vi "LCR Full Advanced Sequence.vi"() -> ()   [LabVIEW 2023]
doc: "Overview: This example demonstrates how to make sweep times faster by using LCR Advanced Sequence functions to change the frequency in a sequence. During the sequence, the channel steps through the predetermined set configurations (frequency in this example) without any interaction with the host system. The advantage of sequencing is that changes from one step in the sequence to the next are deterministic.\nThe program will perform an AC Voltage frequency sweep from Start Frequency to End Frequency. The sweep frequencies are an exponential sequence and the length of each of the sweeps is equal to the value in the Number Of Steps control."
uses:
  <instrlib>/niDCPower/nidcpower.llb/niDCPower Source Mode.ctl
  <instrlib>/niDCPower/nidcpower.llb/niDCPower Wait For Event - Event.ctl
  <instrlib>/niDCPower/nidcpower.llb/niDCPower Sequence Attribute Type.ctl
  <instrlib>/niDCPower/nidcpower.llb/niDCPower Create Advanced Sequence Step With Channels.vi
  <vilib>/Utility/file.llb/Write Delimited Spreadsheet (DBL).vi
panel:
  out "error out":errorcluster
  in  "Hardware timed Instrument Settings":T1(array[cluster])=[{"Instrument Mode"=1062, "LCR:AC Stimulus:Voltage Amplitude"=0.1, "LCR:AC Stimulus:Frequency"=1000.0, "Source:DC Voltage:Voltage Level"=0.0, "Source:DC Voltage:Current Limit"=0.0}, {"Instrument Mode"=1062, "LCR:AC Stimulus:Voltage Amplitude"=0.15, "LCR:AC Stimulus:Frequency"=2000.0, "Source:DC Voltage:Voltage Level"=0.0, "Source:DC Voltage:Current Limit"=0.0}, {"Instrument Mode"=1061, "LCR:AC Stimulus:Voltage Amplitude"=0.0, "LCR:AC Stimulus:Frequency"=0.0, "Source:DC Voltage:Voltage Level"=2.0, "Source:DC Voltage:Current Limit"=1e-06}, {"Instrument Mode"=1061, "LCR:AC Stimulus:Voltage Amplitude"=0.0, "LCR:AC Stimulus:Frequency"=0.0, "Source:DC Voltage:Voltage Level"=4.0, "Source:DC Voltage:Current Limit"=1e-05}, {"Instrument Mode"=1062, "LCR:AC Stimulus:Voltage Amplitude"=0.2, "LCR:AC Stimulus:Frequency"=2000.0, "Source:DC Voltage:Voltage Level"=0.0, "Source:DC Voltage:Current Limit"=0.0}] {"Instrument Mode" items=["SMU PS"=1061, "LCR"=1062, "E-Load"=1154]}
  in  "file path (use dialog)":path
  in  "LCR Short Compensation Enabled":bool
  in  "LCR Open Compensation Enabled":bool
  in  "Impedance Range":dbl=100.0 format="%_6p"
  in  "Cable Length":i32(ring)=1123 items=["0m"=1121, "NI Standard 1m"=1122, "NI Standard 2m"=1123, "NI Standard 4m"=1124, "Custom (Onboard Storage)"=1125, "Custom (As Configured)"=1126, "NI Standard Triaxial 1m"=1139, "NI Standard Triaxial 2m"=1140, "NI Standard Triaxial 4m"=1141]
  in  "LCR Custom Measurement Time Sec":dbl caption="LCR Custom \nMeasurement Time Sec" format="%_3p"
  in  "LCR Measurement Time":i32(ring)=1072 items=["Short"=1071, "Medium"=1072, "Long"=1073, "Custom"=1117]
  in  "LCR DC Bias Source":i32(ring)=1066 items=["Off"=1065, "Voltage"=1066, "Current"=1067]
  in  "Voltage Amplitude RMS":dbl=0.7 format="%_6p"
  out "Impendance vs Frequency":T2(graph) caption="Impedance vs DC Voltage"
  in  "Channel Name":string="0"
  in  "Resource Name":refnum<k15>="Dev1"
  # "Overview: This example demonstrates how to make sweep times faster by using LCR Advanced Sequence functions to change the frequency in a sequence. During the sequence, the channel steps through the predetermined set configurations (frequency in this example) without any interaction with the host system. The advantage of sequencing is that changes from one step in the sequence to the next are deterministic. The program will perform an AC Voltage frequency sweep from Start Frequency to End Frequency. The sweep frequencies are an exponential sequence and the length of each of the sweeps is equal to the value in the Number Of Steps control. \n\nThe Cable Length option of \"Custom (As Configured)\" is not supported in this example. Search ni.com for information about NI power supplies/SMUs and the NI-DCPower API.\n\nRequirements: NI-DCPower\nInstructions:\n1. Select the appropriate instrument in the Resource Name control.\n2. Configure the parameters of the sweeps.\n3. Configure the Cable Length to match your cabling setup.\n4. Run the VI."
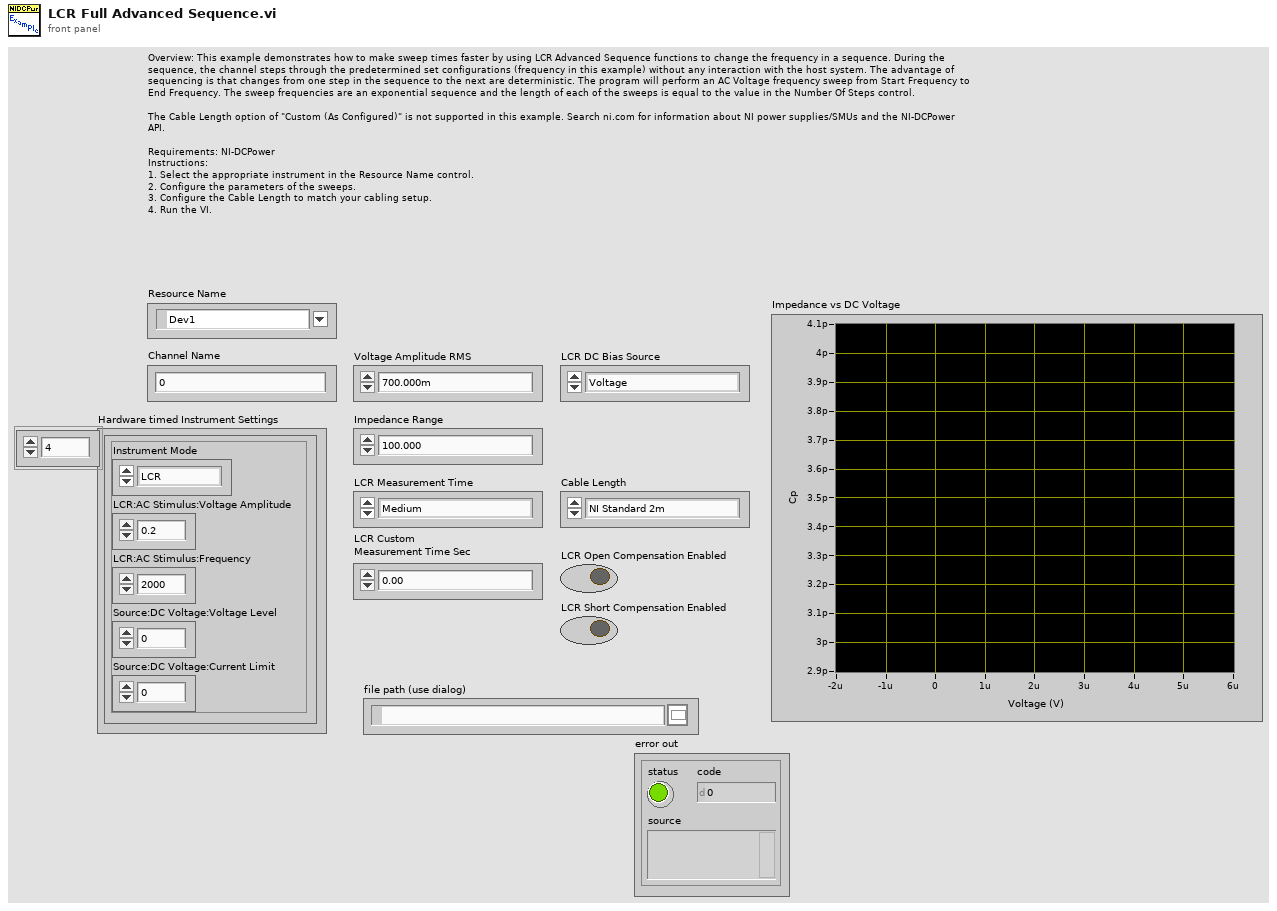
[diagram p1: front panel]
types:
  T1 = cluster{"Instrument Mode":i32, "LCR:AC Stimulus:Voltage Amplitude":dbl, "LCR:AC Stimulus:Frequency":dbl, "Source:DC Voltage:Voltage Level":dbl, "Source:DC Voltage:Current Limit":dbl}[]
  T2 = cluster{"voltage measurements":dbl[], "current measurements":dbl[]}
  T3 = typedef "niDCPower Sequence Attribute Type.ctl" = i32
  T4 = typedef "niDCPower Wait For Event - Event.ctl" = i32
  T5 = typedef "niDCPower Source Mode.ctl" = i32
  T6 = typedef "niDCPower LCR Measurement.ctl" = cluster{"V DC":dbl, "I DC":dbl, "stimulus frequency":dbl, "AC voltage":cdb, "AC current":cdb, "Z":cdb, "Z magnitude":dbl, "Z theta":dbl, "Y":cdb, "Y magnitude":dbl, "Y theta":dbl, "Ls":dbl, "Cs":dbl, "Rs":dbl, "Lp":dbl, "Cp":dbl, "Rp":dbl, "D":dbl, "Q":dbl, "measurement mode":u16, "DC in compliance":bool, "Pad 0":u8, "AC in compliance":bool, "Pad 1":u8, "unbalanced":bool, "Pad 2":u8, "Reserved 1":dbl, "Reserved 2":dbl, "Reserved 3":dbl, "Reserved 4":dbl, "Reserved 5":dbl, "Reserved 6":dbl, "Reserved 7":dbl}
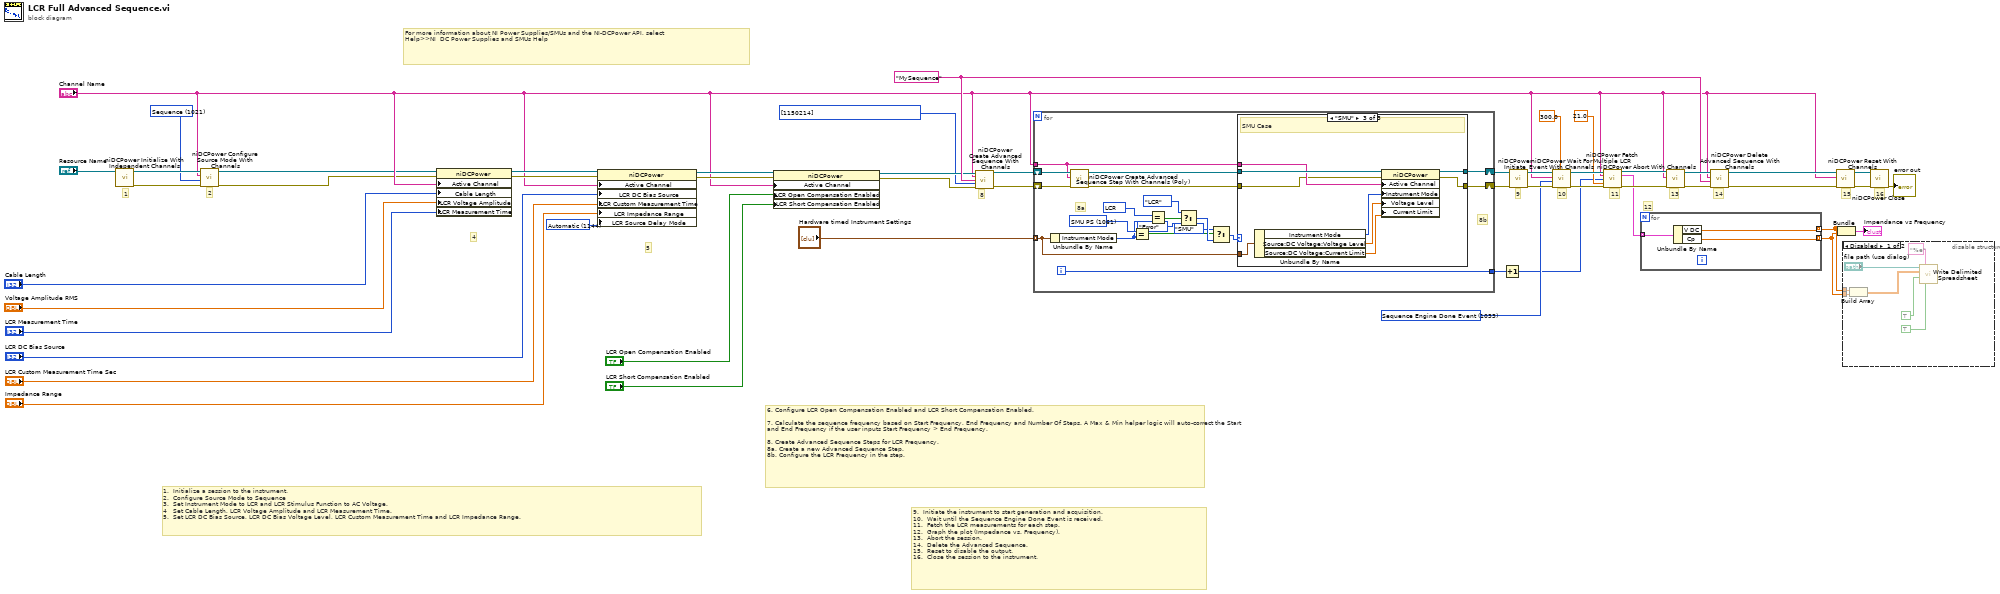
[diagram p0: block diagram]
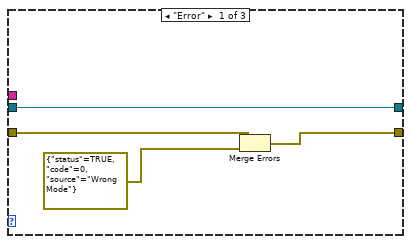
[diagram p3: hidden frame]
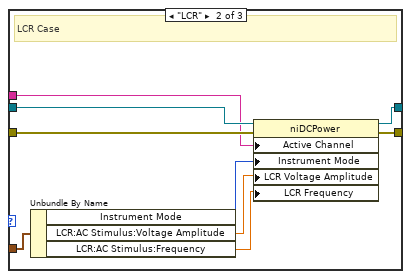
[diagram p4: hidden frame]
diagram:
  w11 = 1144 items=["Automatic"=1144, "Manual"=1145] ("LCR:Source Delay Mode")
  w12 = T3[] [1150214] items=["Source -> Output Function"=1150008, "Source -> Output Enabled"=1250006, "Source -> Output Resistance"=1150061, "Source -> Transient Response"=1150062, "Source -> Custom Transient Response -> Voltage Gain Bandwidth"=1150067, "Source -> Custom Transient Response -> Voltage Compensation Frequency"=1150068, "Source -> Custom Transient Response -> Voltage Pole-Zero Ratio"=1150069, "Source -> Custom Transient Response -> Current Gain Bandwidth"=1150070, "Source -> Custom Transient Response -> Current Compensation Frequency"=1150071, "Source -> Custom Transient Response -> Current Pole-Zero Ratio"=1150072, "Source -> DC Voltage -> Voltage Level"=1250001, "Source -> DC Voltage -> Voltage Level Range"=1150005, "Source -> DC Voltage -> Current Limit"=1250005, "Source -> DC Voltage -> Current Limit High"=1150187, "Source -> DC Voltage -> Current Limit Low"=1150188, "Source -> DC Voltage -> Current Limit Range"=1150004, "Source -> DC Current -> Current Level"=1150009, "Source -> DC Current -> Current Level Range"=1150011, "Source -> DC Current -> Voltage Limit"=1150010, "Source -> DC Current -> Voltage Limit High"=1150185, "Source -> DC Current -> Voltage Limit Low"=1150186, "Source -> DC Current -> Voltage Limit Range"=1150012, "Source -> Pulse Voltage -> Pulse Voltage Level"=1150080, "Source -> Pulse Voltage -> Pulse Bias Voltage Level"=1150082, "Source -> Pulse Voltage -> Pulse Voltage Level Range"=1150084, "Source -> Pulse Voltage -> Pulse Current Limit"=1150081, "Source -> Pulse Voltage -> Pulse Current Limit High"=1150193, "Source -> Pulse Voltage -> Pulse Current Limit Low"=1150194, "Source -> Pulse Voltage -> Pulse Bias Current Limit"=1150083, "Source -> Pulse Voltage -> Pulse Bias Current Limit High"=1150195, "Source -> Pulse Voltage -> Pulse Bias Current Limit Low"=1150196, "Source -> Pulse Voltage -> Pulse Current Limit Range"=1150085, "Source -> Pulse Current -> Pulse Current Level"=1150086, "Source -> Pulse Current -> Pulse Bias Current Level"=1150088, "Source -> Pulse Current -> Pulse Current Level Range"=1150090, "Source -> Pulse Current -> Pulse Voltage Limit"=1150087, "Source -> Pulse Current -> Pulse Voltage Limit High"=1150189, "Source -> Pulse Current -> Pulse Voltage Limit Low"=1150190, "Source -> Pulse Current -> Pulse Bias Voltage Limit"=1150089, "Source -> Pulse Current -> Pulse Bias Voltage Limit High"=1150191, "Source -> Pulse Current -> Pulse Bias Voltage Limit Low"=1150192, "Source -> Pulse Current -> Pulse Voltage Limit Range"=1150091, "Source -> Advanced -> Source Delay"=1150051, "Source -> Advanced -> Pulse Bias Delay"=1150092, "Source -> Advanced -> Pulse On Time"=1150093, "Source -> Advanced -> Pulse Off Time"=1150094, "Source -> Advanced -> OVP Enabled"=1250002, "Source -> Advanced -> OVP Limit"=1250003, "Source -> Advanced -> Compliance Limit Symmetry"=1150184, "Source -> Advanced -> Sequence Step Delta Time"=1150198, "Measurement -> Sense"=1150013, "Measurement -> Aperture Time"=1150058, "Measurement -> Measure Record Length"=1150063, "Measurement -> Advanced -> DC Noise Rejection"=1150066, "Measurement -> Autorange"=1150244, "Measurement -> Advanced -> Autorange Behavior"=1150245, "Measurement -> Advanced -> Autorange Aperture Time Mode"=1150246, "Measurement -> Advanced -> Autorange Minimum Aperture Time"=1150247, "Measurement -> Advanced -> Autorange Minimum Aperture Time Units"=1150248, "Measurement -> Advanced -> Autorange Minimum Current Range"=1150255, "Measurement -> Advanced -> Autorange Minimum Voltage Range"=1150256, "Measurement -> Advanced -> Autorange Threshold Mode"=1150257, "Measurement -> Advanced -> Autorange Maximum Delay After Range Change"=1150322, "LCR -> Instrument Mode"=1150208, "LCR -> Source Delay Mode"=1150315, "LCR -> Measurement Time"=1150218, "LCR -> Custom Measurement Time"=1150258, "LCR -> AC Stimulus -> Function"=1150209, "LCR -> AC Stimulus -> Frequency"=1150210, "LCR -> AC Stimulus -> Voltage Amplitude"=1150211, "LCR -> AC Stimulus -> Current Amplitude"=1150212, "LCR -> AC Stimulus -> Advanced -> Voltage Range"=1150265, "LCR -> AC Stimulus -> Advanced -> Current Range"=1150267, "LCR -> DC Bias -> Source"=1150213, "LCR -> DC Bias -> Voltage Level"=1150214, "LCR -> DC Bias -> Current Level"=1150215, "LCR -> DC Bias -> Advanced -> Voltage Range"=1150266, "LCR -> DC Bias -> Advanced -> Current Range"=1150274, "LCR -> Compensation -> Open -> Enabled"=1150220, "LCR -> Compensation -> Open -> Conductance"=1150261, "LCR -> Compensation -> Open -> Susceptance"=1150262, "LCR -> Compensation -> Short -> Enabled"=1150221, "LCR -> Compensation -> Short -> Resistance"=1150263, "LCR -> Compensation -> Short -> Reactance"=1150264, "LCR -> Compensation -> Load -> Enabled"=1150222, "LCR -> Compensation -> Load -> Measured Resistance"=1150268, "LCR -> Compensation -> Load -> Measured Reactance"=1150269, "LCR -> Compensation -> Load -> Actual Resistance"=1150270, "LCR -> Compensation -> Load -> Actual Reactance"=1150271, "LCR -> Impedance Range -> Impedance Range"=1150217, "LCR -> Impedance Range -> Impedance Autorange"=1150216, "LCR -> Impedance Range -> Advanced -> Impedance Range Source"=1150321, "LCR -> Impedance Range -> Advanced -> Load Resistance"=1150318, "LCR -> Impedance Range -> Advanced -> Load Inductance"=1150319, "LCR -> Impedance Range -> Advanced -> Load Capacitance"=1150320] ("advanced sequence properties")
  w33 = "MySequence" ("sequence name")
  w42 = T4 1033 items=["Source Complete Event"=1030, "Measure Complete Event"=1031, "Sequence Iteration Complete Event"=1032, "Sequence Engine Done Event"=1033] ("event")
  w47 = T5 1021 items=["Single Point"=1020, "Sequence"=1021] ("source mode")
  # "1"
  # "5"
  # "6. Configure LCR Open Compensation Enabled and LCR Short Compensation Enabled.\n\n7. Calculate the sequence frequency based on Start Frequency, End Frequency and Number Of Steps. A Max & Min helper logic will auto-correct the Start and End Frequency if the user inputs Start Frequency > End Frequency.\n\n8. Create Advanced Sequence Steps for LCR Frequency.\n8a. Create a new Advanced Sequence Step.\n8b. Configure the LCR Frequency in the step."
  # "4"
  # "8"
  # "13"
  # "14"
  # "9.  Initiate the instrument to start generation and acquisition.\n10.  Wait until the Sequence Engine Done Event is received.\n11.  Fetch the LCR measurements for each step.\n12.  Graph the plot (Impedance vs. Frequency).\n13.  Abort the session.\n14.  Delete the Advanced Sequence.\n15.  Reset to disable the output.\n16.  Close the session to the instrument."
  # "For more information about NI Power Supplies/SMUs and the NI-DCPower API, select\nHelp>>NI  DC Power Supplies and SMUs Help"
  # "16"
  # "9"
  # "11"
  # "10"
  # "2"
  # "1.  Initialize a session to the instrument.\n2.  Configure Source Mode to Sequence \n3.  Set Instrument Mode to LCR and LCR Stimulus Function to AC Voltage.\n4   Set Cable Length, LCR Voltage Amplitude and LCR Measurement Time. \n5.  Set LCR DC Bias Source, LCR DC Bias Voltage Level, LCR Custom Measurement Time and LCR Impedance Range."
  # "12"
  # "15"
  n1 = call <instrlib>:"niDCPower Initialize With Independent Channels.vi"("resource name"="Resource Name") -> ("error out"=w49:errorcluster, "instrument handle out"=w48:refnum<k15>)  [unwired: 9 in]
  n2 = call <instrlib>:"niDCPower Configure Source Mode With Channels.vi"("error in (no error)"=w49, "source mode"=w47, "channel name"="Channel Name", "instrument handle"=w48) -> ("error out"=w2:errorcluster, "instrument handle out"=w1:refnum<k15>)  [unwired: 6 in]
  n3 = property class="niDCPower"(reference=w1, error in=w2, "Active Channel"="Channel Name", "Cable Length"="Cable Length", "LCR Voltage Amplitude"="Voltage Amplitude RMS", "LCR Measurement Time"="LCR Measurement Time") -> (reference out=w21:refnum<k15>, error out=w20:errorcluster)
  n4 = property class="niDCPower"(reference=w21, error in=w20, "Active Channel"="Channel Name", "LCR DC Bias Source"="LCR DC Bias Source", "LCR Custom Measurement Time"="LCR Custom Measurement Time Sec", "LCR Impedance Range"="Impedance Range", "LCR Source Delay Mode"=w11) -> (reference out=w27:refnum<k15>, error out=w26:errorcluster)
  n5 = property class="niDCPower"(reference=w27, error in=w26, "Active Channel"="Channel Name", "LCR Open Compensation Enabled"="LCR Open Compensation Enabled", "LCR Short Compensation Enabled"="LCR Short Compensation Enabled") -> (reference out=w25:refnum<k15>, error out=w24:errorcluster)
  n6 = call <instrlib>:"niDCPower Create Advanced Sequence With Channels.vi"("instrument handle"=w25, "channel name"="Channel Name", "sequence name"=w33, "advanced sequence properties"=w12, "error in (no error)"=w24) -> ("instrument handle out"=w35:refnum<k15>, "error out"=w34:errorcluster)  [unwired: 9 in]
  n7 = for {
    shift-right: [w68] -> w31
    shift-left: w34 -> [w70]
    tunnel: "Channel Name" -> [w66]
    shift-right: [w67] -> w32
    shift-left: w35 -> [w69]
    tunnel: "Hardware timed Instrument Settings" -> [w63] mode=indexing
    tunnel: [w62] -> w5
    i -> [w62]
    w60 = 1062 items=["SMU PS"=1061, "LCR"=1062, "E-Load"=1154] ("LCR:Instrument Mode")
    w61 = 1061 items=["SMU PS"=1061, "LCR"=1062, "E-Load"=1154] ("LCR:Instrument Mode")
    # "8b"
    # "8a"
    n8 = Unbundle By Name(w63) -> ("Instrument Mode"=w59:i32)
    n9 = call-poly <instrlib>:"niDCPower Create Advanced Sequence Step With Channels (Poly).vi"("error in (no error)"=w70, "channel name"=w66, "instrument handle"=w69) -> ("error out"=w65:errorcluster, "instrument handle out"=w64:refnum<k15>)  [unwired: 7 in]
    n10 = Equal?(x=w61, y=w59) -> (x = y?=w55:bool)
    n11 = Equal?(x=w60, y=w59) -> (x = y?=w58:bool)
    n12 = Select(t=enum16{"LCR", "SMU", "Error"}."LCR", s=w58, f=enum16{"LCR", "SMU", "Error"}."Error" ("t")) -> (s? t:f=w56:enum16{"LCR", "SMU", "Error"})
    n13 = Select(t=enum16{"LCR", "SMU", "Error"}."SMU", s=w55, f=w56) -> (s? t:f=w52:enum16{"LCR", "SMU", "Error"})
    n14 = case shown="\"SMU\"" w52 {
      tunnel: w64 -> [w74 w83 w92]
      tunnel: w65 -> [w71 w82 w89]
      tunnel: [w72 w81 w88] -> w68
      tunnel: [w74 w80 w91] -> w67
      tunnel: w66 -> [_ w79 w90]
      tunnel: w63 -> [_ w78 w87]
      frame "Error" {
        n15 = Merge Errors(w71, errorcluster {"status"=TRUE, "code"=0, "source"="Wrong Mode"} ("error out")) -> (w72:errorcluster)
      }
      frame "LCR" {
        # "LCR Case"
        n16 = Unbundle By Name(w78) -> ("Instrument Mode"=w75:i32, "LCR:AC Stimulus:Voltage Amplitude"=w77:dbl, "LCR:AC Stimulus:Frequency"=w76:dbl)
        n17 = property class="niDCPower"(reference=w83, error in=w82, "Active Channel"=w79, "Instrument Mode"=w75, "LCR Voltage Amplitude"=w77, "LCR Frequency"=w76) -> (reference out=w80:refnum<k15>, error out=w81:errorcluster)
      }
      frame "SMU" {
        # "SMU Case"
        n18 = Unbundle By Name(w87) -> ("Instrument Mode"=w84:i32, "Source:DC Voltage:Voltage Level"=w86:dbl, "Source:DC Voltage:Current Limit"=w85:dbl)
        n19 = property class="niDCPower"(reference=w92, error in=w89, "Active Channel"=w90, "Instrument Mode"=w84, "Voltage Level"=w86, "Current Limit"=w85) -> (reference out=w91:refnum<k15>, error out=w88:errorcluster)
      }
    }
  }
  n20 = Increment(x=w5) -> (x+1=w4:i32)
  n21 = call <instrlib>:"niDCPower Initiate.vi"("error in (no error)"=w31, "instrument handle"=w32) -> ("error out"=w44:errorcluster, "instrument handle out"=w46:refnum<k15>)  [unwired: 2 in, 6 out]
  n22 = call <instrlib>:"niDCPower Wait For Event With Channels.vi"("timeout (10.0)"=300.0, "error in (no error)"=w44, "event"=w42, "channel name"="Channel Name", "instrument handle"=w46) -> ("error out"=w43:errorcluster, "instrument handle out"=w45:refnum<k15>)  [unwired: 5 in]
  n23 = call <instrlib>:"niDCPower Fetch Multiple LCR.vi"("instrument handle"=w45, "channel name"="Channel Name", "count (1)"=w4, "timeout (1.0)"=21.0, "error in (no error)"=w43) -> ("instrument handle out"=w37:refnum<k15>, "measurements"=w30:T6[], "error out"=w39:errorcluster)  [unwired: 7 in, 1 out]
  n24 = for {
    tunnel: w30 -> [w95] mode=indexing
    tunnel: [w94] -> w9 mode=indexing
    tunnel: [w93] -> w8 mode=indexing
    n25 = Unbundle By Name(w95) -> ("V DC"=w94:dbl, "Cp"=w93:dbl)
  }
  n26 = call <instrlib>:"niDCPower Abort With Channels.vi"("error in (no error)"=w39, "channel name"="Channel Name", "instrument handle"=w37) -> ("error out"=w38:errorcluster, "instrument handle out"=w36:refnum<k15>)  [unwired: 7 in]
  n27 = call <instrlib>:"niDCPower Delete Advanced Sequence With Channels.vi"("error in (no error)"=w38, "sequence name"=w33, "channel name"="Channel Name", "instrument handle"=w36) -> ("error out"=w41:errorcluster, "instrument handle out"=w40:refnum<k15>)  [unwired: 6 in]
  n28 = call <instrlib>:"niDCPower Reset With Channels.vi"("error in (no error)"=w41, "channel name"="Channel Name", "instrument handle"=w40) -> ("error out"=w50:errorcluster, "instrument handle out"=w51:refnum<k15>)  [unwired: 7 in]
  n29 = Bundle(w9, w8) -> (→"Impendance vs Frequency":cluster{dbl[], dbl[]})  [unwired: 1 out]
  n30 = disable-structure shown="Disabled" {
    disable-tunnel: w9 -> [w102 _]
    disable-tunnel: w8 -> [w101 _]
    frame Disabled {
      n31 = Build Array(w102, w101) -> (w100:dbl[][])
      n32 = call-poly <vilib>:"Write Delimited Spreadsheet.vi"("file path (dialog if empty)"="file path (use dialog)", "format (%.3f)"="%e", "2D data"=w100, "append to file? (new file:F)"=TRUE, "transpose? (no:F)"=TRUE) -> ()  [unwired: 9 in, 2 out]
    }
    frame Enabled {
    }
  }
  n33 = call <instrlib>:"niDCPower Close.vi"("error in (no error)"=w50, "instrument handle"=w51) -> ("error out"=→"error out":errorcluster)  [unwired: 9 out]
